vi "Datasheet Parameter String.vi"(1 "params":T1) -> (0 "url-encoded param string":string)   [LabVIEW 2011]
doc: "Builds a URL-encoded parameter list from a keyed array. Use this VI to build the parameters for a link to a CGI application."
uses:
  Addons/internet/utils/keyedarr.llb/Keyed Array.ctl
panel:
  out "length":i32
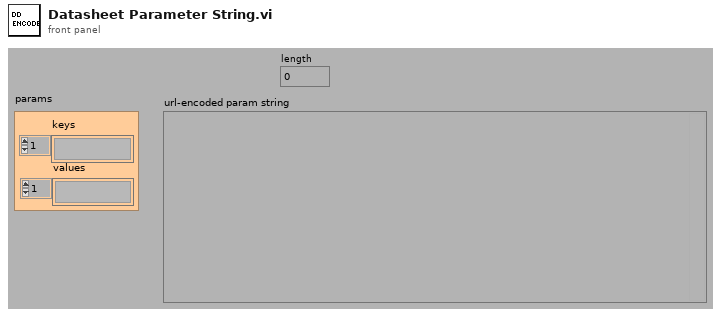
[diagram p1: front panel]
types:
  T1 = typedef "Keyed Array.ctl" = cluster{"keys":string[], "values":string[]}
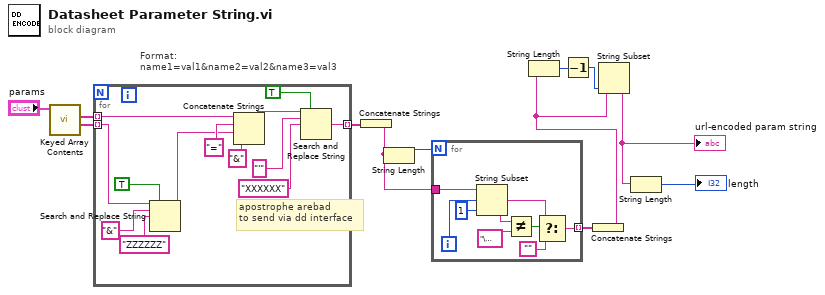
[diagram p0: block diagram]
diagram:
  # "Format:\nname1=val1&name2=val2&name3=val3"
  n1 = call "Keyed Array Contents.vi"("array in"="params") -> ("values"=w10:string[], "keys"=w11:string[])  [unwired: 5 out]
  n2 = for {
    tunnel: w11 -> [w23] mode=indexing
    tunnel: w10 -> [w14] mode=indexing
    tunnel: [w18] -> w7 mode=indexing
    # "apostrophe arebad\nto send via dd interface"
    n3 = Search and Replace String(replace all?=TRUE ("replace all? (F)"), input string=w14, search string="&", replace string="ZZZZZZ" ("replace string (\"\")")) -> (result string=w13:string)  [unwired: 1 in, 6 out]
    n4 = Concatenate Strings(w23, "=", w13, "&") -> (w22:string)
    n5 = Search and Replace String(replace all?=TRUE ("replace all? (F)"), input string=w22, search string="'", replace string="XXXXXX" ("replace string (\"\")")) -> (result string=w18:string)  [unwired: 1 in, 6 out]
  }
  n6 = Concatenate Strings(w7) -> (w2:string)
  n7 = String Length(string=w2) -> (length=w4:i32)
  n8 = for {
    N: w4 -> [_]
    tunnel: w2 -> [w33]
    tunnel: [w28] -> w3 mode=indexing
    i -> [w32]
    n9 = String Subset(string=w33, offset (0)=w32, length (rest)=1 ("length (rest)")) -> (substring=w29:string)
    n10 = Not Equal?(x=w29, y="\u0000" ("search string")) -> (x != y?=w26:bool)
    n11 = Select(t=w29, s=w26, f="") -> (s? t:f=w28:string)
  }
  n12 = Concatenate Strings(w3) -> (w1:string)
  n13 = String Length(string=w1) -> (length=w9:i32)
  n14 = Decrement(x=w9) -> (x-1=w8:i32)
  n15 = String Subset(string=w1, length (rest)=w8) -> (substring=w5:string)  [unwired: 1 out]
  "url-encoded param string" <- w5
  n16 = String Length(string=w5) -> (length=→"length":i32)
